vi "IMAQ FPGA CXP U64x4 to U8x32.vi"(11 "Pixel Data U64x4":u64[](array[numeric])=[0, 0, 0, 0]) -> (3 "Pixel Data Out U8x32":u8[](array[numeric]))   [LabVIEW 2020]
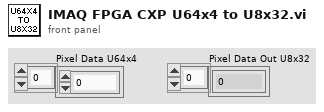
[diagram p1: front panel]
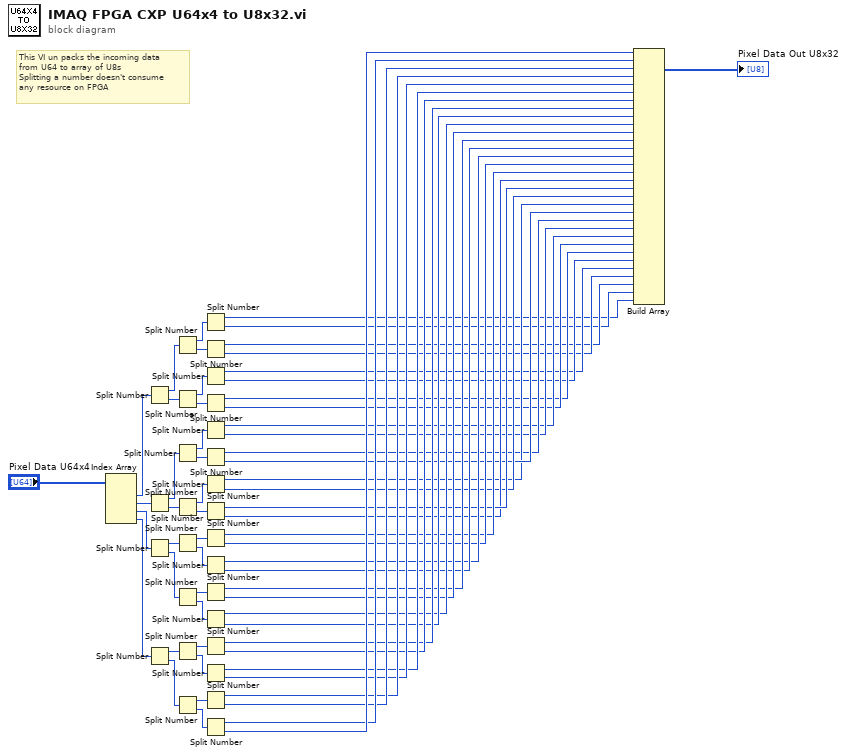
[diagram p0: block diagram]
diagram:
  # "This VI un packs the incoming data\nfrom U64 to array of U8s\nSplitting a number doesn't consume\nany resource on FPGA"
  n1 = Index Array(array="Pixel Data U64x4") -> (element #1=w61:u64, element #2=w60:u64, element #3=w59:u64, element #4=w58:u64)  [unwired: 4 in]
  n2 = Split Number(x=w61) -> (hi(x)=w57:u32, lo(x)=w56:u32)
  n3 = Split Number(x=w60) -> (hi(x)=w55:u32, lo(x)=w54:u32)
  n4 = Split Number(x=w59) -> (hi(x)=w53:u32, lo(x)=w52:u32)
  n5 = Split Number(x=w58) -> (hi(x)=w51:u32, lo(x)=w50:u32)
  n6 = Split Number(x=w57) -> (hi(x)=w49:u16, lo(x)=w48:u16)
  n7 = Split Number(x=w56) -> (hi(x)=w47:u16, lo(x)=w46:u16)
  n8 = Split Number(x=w55) -> (hi(x)=w45:u16, lo(x)=w44:u16)
  n9 = Split Number(x=w54) -> (hi(x)=w43:u16, lo(x)=w42:u16)
  n10 = Split Number(x=w53) -> (hi(x)=w41:u16, lo(x)=w40:u16)
  n11 = Split Number(x=w52) -> (hi(x)=w39:u16, lo(x)=w38:u16)
  n12 = Split Number(x=w51) -> (hi(x)=w37:u16, lo(x)=w36:u16)
  n13 = Split Number(x=w50) -> (hi(x)=w35:u16, lo(x)=w34:u16)
  n14 = Split Number(x=w49) -> (hi(x)=w1:u8, lo(x)=w2:u8)
  n15 = Split Number(x=w48) -> (hi(x)=w3:u8, lo(x)=w4:u8)
  n16 = Split Number(x=w47) -> (hi(x)=w5:u8, lo(x)=w6:u8)
  n17 = Split Number(x=w46) -> (hi(x)=w7:u8, lo(x)=w8:u8)
  n18 = Split Number(x=w45) -> (hi(x)=w9:u8, lo(x)=w10:u8)
  n19 = Split Number(x=w44) -> (hi(x)=w11:u8, lo(x)=w13:u8)
  n20 = Split Number(x=w43) -> (hi(x)=w12:u8, lo(x)=w14:u8)
  n21 = Split Number(x=w42) -> (hi(x)=w16:u8, lo(x)=w15:u8)
  n22 = Split Number(x=w41) -> (hi(x)=w17:u8, lo(x)=w18:u8)
  n23 = Split Number(x=w40) -> (hi(x)=w19:u8, lo(x)=w20:u8)
  n24 = Split Number(x=w39) -> (hi(x)=w21:u8, lo(x)=w22:u8)
  n25 = Split Number(x=w38) -> (hi(x)=w24:u8, lo(x)=w25:u8)
  n26 = Split Number(x=w37) -> (hi(x)=w26:u8, lo(x)=w27:u8)
  n27 = Split Number(x=w36) -> (hi(x)=w28:u8, lo(x)=w29:u8)
  n28 = Split Number(x=w35) -> (hi(x)=w30:u8, lo(x)=w31:u8)
  n29 = Split Number(x=w34) -> (hi(x)=w32:u8, lo(x)=w33:u8)
  n30 = Build Array(w33, w32, w31, w30, w29, w28, w27, w26, w25, w24, w22, w21, w20, w19, w18, w17, w15, w16, w14, w12, w13, w11, w10, w9, w8, w7, w6, w5, w4, w3, w2, w1) -> (→"Pixel Data Out U8x32":u8[])
